vi "AI-loop.vi"(8 "错误输入（无错误）":errorcluster, 11 "Status":T1 {"Setting"."X Pos." scale=-2.0..2.0; "Setting"."Y Pos." scale=-2.0..2.0}) -> (0 "Error out":errorcluster caption="错误输入（无错误）")   [LabVIEW 2013]
uses:
  init & communication/init-status.ctl
  init & communication/Setting.ctl
  init & communication/event-package.ctl
  init & communication/Event1.ctl
  init & communication/data-package.ctl
  init & communication/Event.ctl
  <vilib>/DAQmx/read.llb/DAQmx Read (Analog 1D DBL 1Chan NSamp).vi
  <vilib>/DAQmx/create/channels.llb/DAQmx Create Channel (AI-Voltage-Basic).vi
  <vilib>/DAQmx/configure/timing.llb/DAQmx Timing (Sample Clock).vi
  <vilib>/DAQmx/configure/trigger.llb/DAQmx Start Trigger (Digital Edge).vi
  <vilib>/DAQmx/miscellaneous.llb/DAQmx Fill In Error Info.vi
  <resource>/objmgr/daqmx.rc
panel:
  out "NoS per Channell":i32
  out "loop (frame) #":i32
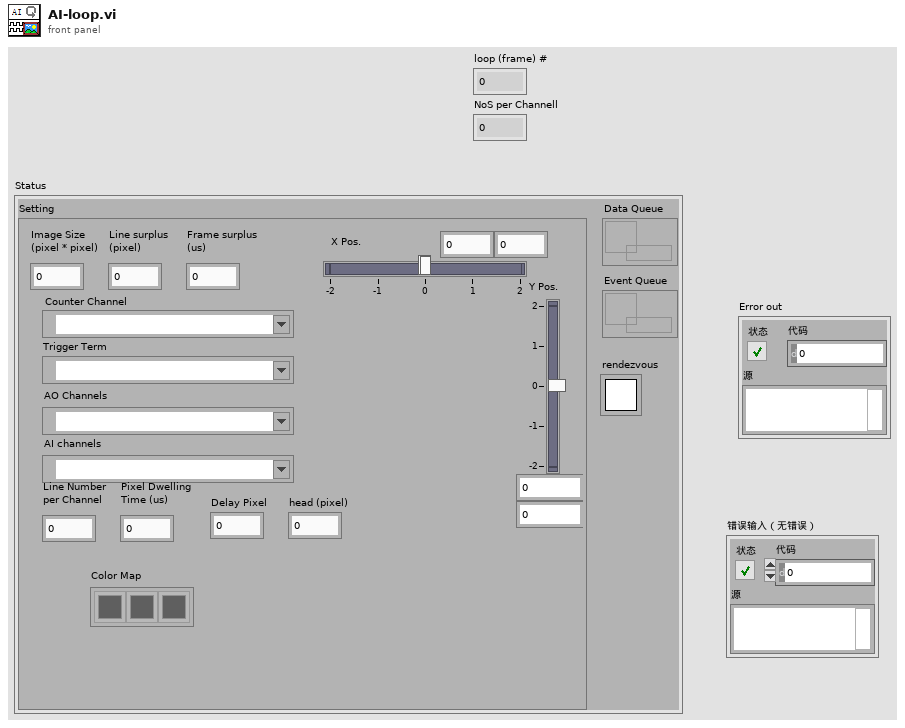
[diagram p1: front panel]
types:
  T1 = typedef "init-status.ctl" = cluster{"Setting":T2, "Event Queue":refnum<queue>, "Data Queue":refnum<queue>, "rendezvous":T3}
  T2 = typedef "Setting.ctl" = cluster{"Image Size\n(pixel * pixel)":i32, "Counter Channel":tag, "Trigger Term":tag, "AO Channels":tag, "Y Pos.":cluster{dbl, dbl}, "X Pos.":cluster{dbl, dbl}, "Line surplus\n(pixel)":i32, "Frame surplus\n(us)":i32, "AI channels":tag, "Line Number\nper Channel":i32, "Delay Pixel":i32, "Pixel Dwelling\nTime (us)":i32, "Color Map":u32[], "head (pixel)":i32}
  T3 = typedef "Rendezvous RefNum" = refnum<k1>
  T4 = typedef "data-package.ctl" = cluster{"Event":T5, "Data":dbl[], "line #":i32}
  T5 = typedef "Event.ctl" = u16
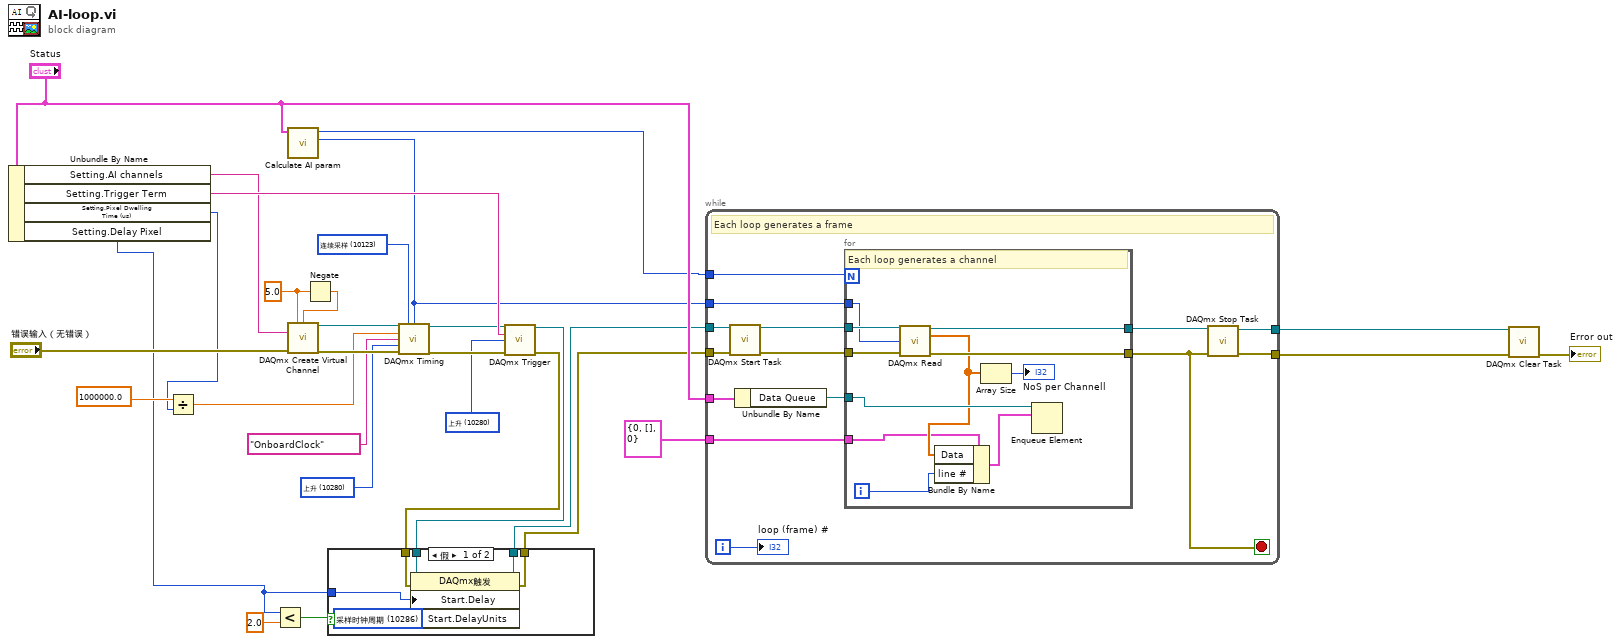
[diagram p0: block diagram]
diagram:
  w18 = 10280 items=["上升"=10280, "下降"=10171] ("edge")
  w21 = 10123 items=["有限采样"=10178, "连续采样"=10123, "硬件定时单点"=12522] ("sample mode")
  w22 = 10280 items=["上升"=10280, "下降"=10171] ("active edge")
  w27 = 5.0
  n1 = Unbundle By Name("Status") -> ("Setting.AI channels"=w28:tag, "Setting.Trigger Term"=w29:tag, "Setting.Pixel Dwelling\nTime (us)"=w10:i32, "Setting.Delay Pixel"=w5:i32)
  n2 = Divide(x=1000000.0 ("rate"), y=w10) -> (x/y=w9:dbl)
  n3 = Less?(x=w5, y=2.0) -> (x < y?=w6:bool)
  n4 = call "Calculate AI param.vi"("Status"="Status") -> ("# samples per channel"=w12:i32, "# channels per frame"=w13:i32)  [unwired: 9 in]
  n5 = Negate(x=w27) -> (-x=w26:dbl)
  n6 = call-poly <vilib>:"DAQmx Create Virtual Channel.vi"("maximum value"=w27, "minimum value"=w26, "physical channels"=w28, "error in"="错误输入（无错误）") -> ("task out"=w25:refnum<k21>, "error out"=w24:errorcluster)  [unwired: 10 in]
  n7 = call-poly <vilib>:"DAQmx Timing.vi"("task/channels in"=w25, "sample mode"=w21, "samples per channel"=w12, "rate"=w9, "source"=tag "OnboardClock", "active edge"=w22, "error in"=w24) -> ("task out"=w20:refnum<k21>, "error out"=w19:errorcluster)  [unwired: 7 in]
  n8 = call-poly <vilib>:"DAQmx Trigger.vi"("task/channels in"=w20, "source"=w29, "edge"=w18, "error in"=w19) -> ("task out"=w4:refnum<k21>, "error out"=w3:errorcluster)  [unwired: 10 in]
  n9 = case shown="假" w6 {
    tunnel: w4 -> [w36 w38]
    tunnel: [w35 w38] -> w2
    tunnel: w3 -> [w34 w37]
    tunnel: [w33 w37] -> w1
    tunnel: w5 -> [w32 _]
    frame False {
      w31 = 10286 items=["采样时钟周期"=10286, "秒"=10364, "时钟滴答"=10304] ("Start.DelayUnits")
      n10 = property class="DAQmx触发"(reference=w36, error in=w34, "Start.Delay"=w32, "Start.DelayUnits"=w31) -> (reference out=w35:refnum<k21>, error out=w33:errorcluster)
    }
    frame True {
    }
  }
  n11 = while {
    tunnel: w2 -> [w45]
    tunnel: w1 -> [w42]
    tunnel: [w48] -> w15
    tunnel: [w47] -> w16
    tunnel: "Status" -> [w52]
    tunnel: w13 -> [w41]
    tunnel: w12 -> [w40]
    tunnel: T4 {"Event"=0, "Data"=[], "line #"=0} ("Data Package") -> [w39]
    i -> [w50]
    stop <- w49 stop-if-true
    # "Each loop generates a frame"
    n12 = call <vilib>:"DAQmx Start Task.vi"("task/channels in"=w45, "error in"=w42) -> ("task out"=w44:refnum<k21>, "error out"=w43:errorcluster)  [unwired: 12 in]
    n13 = Unbundle By Name(w52) -> ("Data Queue"=w51:refnum<queue>)
    n14 = for {
      N: w41 -> [_]
      tunnel: w44 -> [w63]
      tunnel: w43 -> [w62]
      tunnel: [w61] -> w49
      tunnel: [w60] -> w46
      tunnel: w51 -> [w59]
      tunnel: w40 -> [w56]
      tunnel: w39 -> [w53]
      i -> [w57]
      # "Each loop generates a channel"
      n15 = call-poly <vilib>:"DAQmx Read.vi"("task/channels in"=w63, "number of samples per channel"=w56, "error in"=w62) -> ("task out"=w60:refnum<k21>, "data"=w55:dbl[], "error out"=w61:errorcluster)  [unwired: 10 in]
      n16 = Bundle By Name(cluster=w53, "Data"=w55, "line #"=w57) -> (w58:T4)
      n17 = Array Size(array=w55) -> (size(s)=→"NoS per Channell":i32)
      n18 = Enqueue Element(queue=w59, element=w58) -> ()  [unwired: 2 in, 3 out]
    }
    n19 = call <vilib>:"DAQmx Stop Task.vi"("task/channels in"=w46, "error in"=w49) -> ("task out"=w47:refnum<k21>, "error out"=w48:errorcluster)  [unwired: 12 in]
    "loop (frame) #" <- w50
  }
  n20 = call <vilib>:"DAQmx Clear Task.vi"("task in"=w16, "error in"=w15) -> ("error out"=→"Error out":errorcluster)  [unwired: 13 in]
